vi "Scale Pump Head-Flow Curves.vi"(6 "speeds":dbl[](array[numeric]), 10 "head":dbl[](array[numeric]), 11 "flow":dbl[](array[numeric])) -> (3 "head-flow curves":cluster{dbl[], dbl[]}[](array[cluster]))   [LabVIEW 2020]
doc: "Scale a pump head-flow curve to different speeds according to the scaling relationships for geometrically similar pumps; i.e. flow2 = (speed2 / speed1) * flow1 and head2 = (speed2 / speed1)^2 * head1. The first speed in the array is assumed to be the speed of the provided head-flow curve."
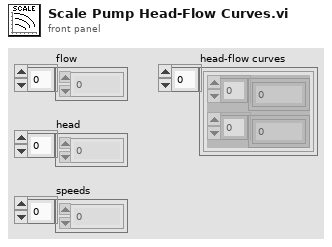
[diagram p1: front panel]
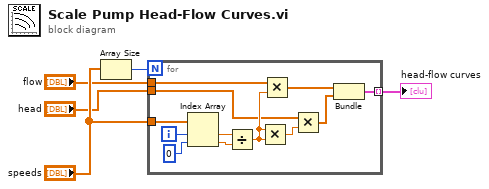
[diagram p0: block diagram]
diagram:
  n1 = Array Size(array="speeds") -> (size(s)=w5:i32)
  n2 = for {
    N: w5 -> [_]
    tunnel: "speeds" -> [w17]
    tunnel: "flow" -> [w12]
    tunnel: "head" -> [w10]
    tunnel: [w6] -> w3 mode=indexing
    i -> [w15]
    n3 = Index Array(array=w17, index #1=w15, index #2=0 ("index")) -> (element #1=w14:dbl, element #2=w13:dbl)
    n4 = Divide(x=w14, y=w13) -> (x/y=w11:dbl)
    n5 = Multiply(x=w11, y=w11) -> (x*y=w9:dbl)
    n6 = Multiply(x=w12, y=w11) -> (x*y=w7:dbl[])
    n7 = Multiply(x=w10, y=w9) -> (x*y=w8:dbl[])
    n8 = Bundle(w7, w8) -> (w6:cluster{dbl[], dbl[]})  [unwired: 1 in]
  }
  "head-flow curves" <- w3
